vi "AfficherLivraison.vi"() -> (0 "Result Set":string[][](table), 1 "?":string[](array[string]))   [LabVIEW 2024]
uses:
  <vilib>/drjdpowell/SQLite Library/SQL Statement/SQL Statement.lvclass/SQL Statement.ctl
  <vilib>/drjdpowell/SQLite Library/SQL Connection/Open (string).vi
  <vilib>/drjdpowell/SQLite Library/SQL Connection/Execute SQL.vi
  <vilib>/drjdpowell/SQLite Library/SQL Statement/Error Message.vi
  <vilib>/drjdpowell/SQLite Library/SQL Connection/Connection.lvclass
  <vilib>/drjdpowell/SQLite Library/SQLite.lvlib
panel:
  # "Liste des livraisons"
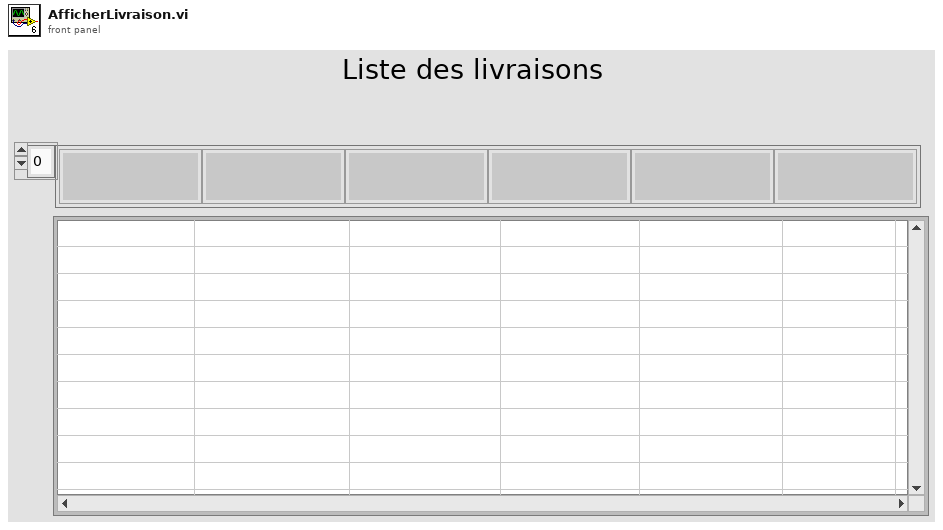
[diagram p1: front panel]
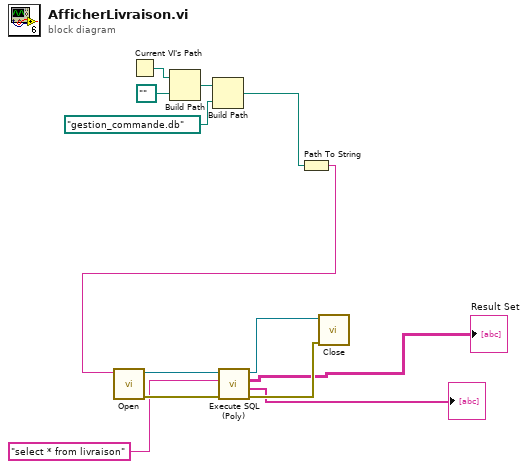
[diagram p0: block diagram]
diagram:
  n1 = Current VI's Path() -> (path=w9:path)
  n2 = Build Path(base path=w9, name or relative path=path "..") -> (appended path=w6:path)
  n3 = Build Path(base path=w6, name or relative path=path "gestion_commande.db" ("Filename")) -> (appended path=w5:path)
  n4 = Path To String(path=w5) -> (string=w4:string)
  n5 = call-poly <vilib>:"Open.vi"("db file"=w4) -> ("error out"=w12:errorcluster, "SQLite Connection"=w13:refnum<class "Connection.lvclass">)  [unwired: 9 in]
  n6 = call-poly <vilib>:"Execute SQL (Poly).vi"("error in (no error)"=w12, "SQL"="select * from livraison", "SQLite Connection in"=w13) -> ("error out"=w11:errorcluster, "Column Names"=→"?":string[], "Result Set"=→"Result Set":string[][], "SQLite Connection"=w10:refnum<class "Connection.lvclass">)  [unwired: 5 in]
  n7 = call-dynamic "Close.vi"("error in (no error)"=w11, "SQLite Connection in"=w10) -> ()  [unwired: 9 in, 1 out]
